vi "Set Temperature.vi"(8 "error in (no error)":errorcluster, 10 "On/Off":bool, 11 "Process Settings in":refnum<class "Process Settings.lvclass">) -> (0 "error out":errorcluster, 3 "Process Settings out":refnum<class "Process Settings.lvclass">)   [LabVIEW 2017, in "Expansion.lvclass"]
uses:
  Expansion.lvclass
  Process Settings/Process Settings.lvclass
  Hardware Settings/Type Defs/Hardware Types.ctl
  Process Settings/Type Defs/Item.ctl
  Process Settings/Process Settings.lvclass/Process Settings.ctl
  Process Settings/Accessors/Read Hardware Settings.vi
  Hardware Settings/Hardware Settings.lvclass
  Hardware Settings/Hardware Types/Generic/Generic Hardware.lvclass
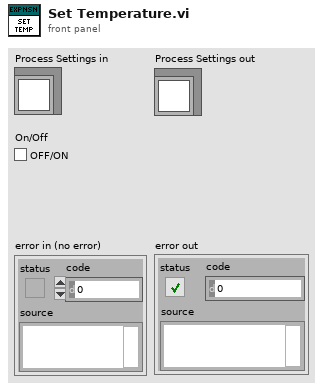
[diagram p1: front panel]
types:
  T1 = typedef "Process Settings.lvclass/Item.ctl" = enum16{"", "sheet temperature setpoint", "sheet heating time", "temp element setpoint", "chamber pressure setpoint", "saturation time", "chamber pressure valve setpoint"}
  T2 = typedef "Hardware Settings.lvclass/Hardware Types.ctl" = enum16{"Tank Chamber Pressure and Temperature", "Tank Valve Controls", "Motor On/Off and Direction Control", "Limit Switches", "IR Temperature", "Pneumatic Cylinder Actuation", "Expansion Temperature Setpoint"}
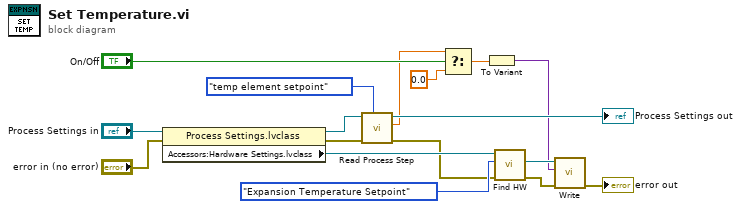
[diagram p0: block diagram]
diagram:
  n1 = property class="Process Settings.lvclass"(reference="Process Settings in", error in="error in (no error)") -> (reference out=w10:refnum<class "Process Settings.lvclass">, error out=w8:errorcluster, "Accessors:Hardware Settings.lvclass"=w11:refnum<class "Hardware Settings.lvclass">)
  n2 = call "Read Process Step.vi"("Item"=Item."temp element setpoint", "error in (no error)"=w8, "Process Settings in"=w10) -> ("error out"=w7:errorcluster, "Value"=w2:dbl, "Process Settings out"=→"Process Settings out":refnum<class "Process Settings.lvclass">)  [unwired: 5 in, 1 out]
  n3 = Select(t=w2, s="On/Off", f=0.0) -> (s? t:f=w1:dbl)
  n4 = To Variant(anything=w1) -> (Variant=w5:variant)
  n5 = call "Find HW.vi"("error in (no error)"=w7, "HW Item"=Hardware_Types."Expansion Temperature Setpoint", "Hardware Settings in"=w11) -> ("error out"=w17:errorcluster, "Selected Hardware Out"=w16:refnum<class "Generic Hardware.lvclass">)  [unwired: 6 in, 1 out]
  n6 = call-dynamic "Write.vi"("error in (no error)"=w17, "Input"=w5, "Generic Hardware in"=w16) -> ("error out"=→"error out":errorcluster)  [unwired: 7 in, 1 out]
